vi "Initialize AO.vi"(8 "error in (no error)":errorcluster, 9 "AO Channel Setting":T1={"AO Channel name"=[], "output terminal configuration"=enum."RSE", "minimum value"=-10.0, "maximum value"=10.0, "units"=enum."Volts", "name to assign"=[]} {"maximum value" format="%0.2f"; "minimum value" format="%0.2f"}, 10 "DAQ Type":enum16{"Hardware", "Simulation"}(ring), 11 "PXIe 6363 in":refnum<class "PXIe 6363.lvclass">) -> (0 "error out":errorcluster, 3 "PXIe 6363 out":refnum<class "PXIe 6363.lvclass">)   [LabVIEW 2016, in "DAQ Hardware.lvlib" / "PXIe 6363.lvclass"]
uses:
  PXIe 6363.lvclass
  AO Channel Setting.ctl
  PXIe 6363.lvclass/PXIe 6363.ctl
  DAQ Hardware.lvlib
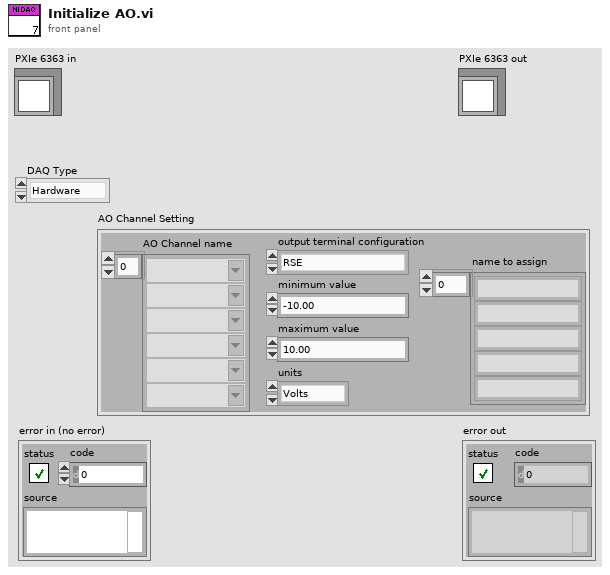
[diagram p1: front panel]
types:
  T1 = typedef "DAQ Hardware.lvlib/AO Channel Setting.ctl" = cluster{"AO Channel name":string[], "output terminal configuration":enum16{"RSE", "NRSE", "Differential"}, "minimum value":dbl, "maximum value":dbl, "units":enum16{"Volts"}, "name to assign":string[]}
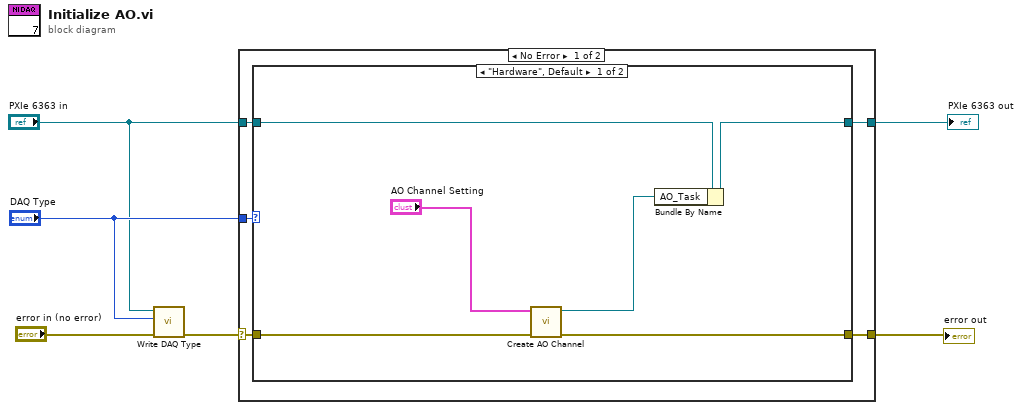
[diagram p0: block diagram]
diagram:
  n1 = call-dynamic "Write DAQ Type.vi"("error in (no error)"="error in (no error)", "DAQ Type"="DAQ Type", "PXIe 6363 in"="PXIe 6363 in") -> ("error out"=w5:errorcluster)  [unwired: 7 in, 1 out]
  n2 = case shown="No Error" w5 {
    selector: w5 -> [w11 w20]
    tunnel: "DAQ Type" -> [w10 _]
    tunnel: [w9 w20] -> w3
    tunnel: "PXIe 6363 in" -> [w8 w21]
    tunnel: [w7 w21] -> w1
    frame No Error {
      n3 = case shown="\"Hardware\", Default" w10 {
        tunnel: w11 -> [w17 w18]
        tunnel: [w16 w18] -> w9
        tunnel: w8 -> [w15 w19]
        tunnel: [w14 w19] -> w7
        frame "Hardware", Default {
          n4 = call "Create AO Channel.vi"("error in (no error)"=w17, "AO Setting"="AO Channel Setting") -> ("error out"=w16:errorcluster, "AO Task"=w13:refnum<k21>)  [unwired: 8 in]
          n5 = Bundle By Name(cluster=w15, "AO_Task"=w13) -> (w14:refnum<class "PXIe 6363.lvclass">)
        }
        frame "Simulation" {
        }
      }
    }
    frame Error {
    }
  }
  "error out" <- w3
  "PXIe 6363 out" <- w1
